vi "closePort.vi"(8 "error in (no error)":errorcluster) -> (0 "error out":errorcluster)   [LabVIEW 2015, in "TPVG_DLL.lvlib"]
doc: "------------------------------------------\nAuthor: Dang Lam\nEmail: danglamtd@gmail.com"
uses:
  TPVG_DLL.lvlib
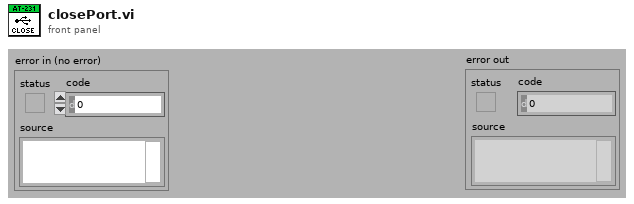
[diagram p1: front panel]
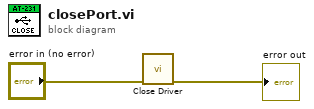
[diagram p0: block diagram]
diagram:
  n1 = call "Close Driver.vi"("error in (no error)"="error in (no error)") -> ("error out"=→"error out":errorcluster)  [unwired: 10 in]
